vi "THD_MSA_for_teststand_Seq.vi"(6 "Sound_Pressure(dB SPL)":dbl=94.0502, 8 "error in":errorcluster, 9 "Std_Deviation_Thresold":dbl=0.04, 10 "frequency list Input":T6(array[cluster])=[{"frequency [Hz]"=1000.0, "amplitude [V]"=0.373}] {"amplitude [V]" format="%.6f"; "frequency [Hz]" format="%.2f"}, 11 "Peiker_Stepped Sweep Settings":T1={"Input Settings"={"IEPE min time to settle [s]"=0.0, "Responce Channel Settings"={"DSA response channel settings"={"coupling"=10045, "enable IEPE excitation"=FALSE, "IEPE current [mA]"=4.0}, "response channel info"={"sensor sensitivity"=200.0, "engineering units"=2, "dB reference"=2e-05, "custom label"="EU", "weighting filter"=0, "pregain"=0.0}, "AI response settings"={"response channel"="SOUNDACQ/ai1", "max value [V]"=10.0, "min value [V]"=-10.0, "terminal configuration"=-1}}, "Stimulus Channel Settings"={"AI stimulus settings"={"stimulus channel"="SOUNDACQ/ai0", "max value [V]"=10.0, "min value [V]"=-10.0, "terminal configuration"=-1}, "DSA stimulus channel settings"={"coupling"=10045, "enable IEPE excitation"=TRUE, "IEPE current [mA]"=4.0}, "stimulus channel info"={"sensor sensitivity"=11.4, "engineering units"=2, "dB reference"=2e-05, "custom label"="EU", "weighting filter"=0, "pregain"=0.0}}}, "Output Settings"={"AO source settings"={"excitation channel"="SOUNDACQ/ao0", "max value [V]"=10.0, "min value [V]"=-10.0, "terminal configuration"=-1}}} {"Output Settings"."AO source settings"."terminal configuration" items=["Default"=-1, "RSE"=10083, "Differential"=10106, "Pseudodifferential"=12529]; "Output Settings"."AO source settings"."min value [V]" format="%0.2f"; "Output Settings"."AO source settings"."max value [V]" format="%0.2f"; "Input Settings"."Stimulus Channel Settings"."stimulus channel info"."pregain" format="%.2f"; "Input Settings"."Stimulus Channel Settings"."stimulus channel info"."weighting filter" items=["Linear", "A-weighting", "B-weighting", "C-weighting", "ITU-R 468-4", "Dolby", "CCITT", "C-message", "Wb", "Wc", "Wd", "We", "Wf", "Wh", "Wj", "Wk", "Wm", "AES17 20 kHz lowpass", "AES17 40 kHz lowpass", "AES17 20 kHz highpass", "AES17 40 kHz highpass"]; "Input Settings"."Stimulus Channel Settings"."stimulus channel info"."dB reference" format="%^.1e"; "Input Settings"."Stimulus Channel Settings"."stimulus channel info"."engineering units" items=["custom..."=0, "V"=1, "A"=21, "C"=30, "pC"=31, "s"=32, "-"=29, "Pa"=2, "N"=20, "g"=3, "m/s^2"=4, "m/s"=5, "m"=6, "mm/s"=12, "mm"=13, "micron/s"=14, "micron"=15, "in/s^2"=7, "in/s"=8, "in"=9, "mil/s"=10, "mil"=11, "rad/s^2"=16, "rad/s"=17, "rad"=18, "deg/s^2"=26, "deg/s"=27, "deg"=28, "RPM"=22, "cycle/s^2"=23, "Hz"=24, "cycle"=25, "strain"=19]; "Input Settings"."Stimulus Channel Settings"."stimulus channel info"."sensor sensitivity" format="%#_5f"; "Input Settings"."Stimulus Channel Settings"."DSA stimulus channel settings"."IEPE current [mA]" format="%.1f"; "Input Settings"."Stimulus Channel Settings"."DSA stimulus channel settings"."coupling" items=["AC"=10045, "DC"=10050, "GND"=10066]; "Input Settings"."Stimulus Channel Settings"."AI stimulus settings"."terminal configuration" items=["Default"=-1, "RSE"=10083, "NRSE"=10078, "Differential"=10106, "Pseudodifferential"=12529]; "Input Settings"."Stimulus Channel Settings"."AI stimulus settings"."min value [V]" format="%.2f"; "Input Settings"."Stimulus Channel Settings"."AI stimulus settings"."max value [V]" format="%.2f"; "Input Settings"."Responce Channel Settings"."AI response settings"."terminal configuration" items=["Default"=-1, "RSE"=10083, "NRSE"=10078, "Differential"=10106, "Pseudodifferential"=12529]; "Input Settings"."Responce Channel Settings"."AI response settings"."min value [V]" format="%.2f"; "Input Settings"."Responce Channel Settings"."AI response settings"."max value [V]" format="%.2f"; "Input Settings"."Responce Channel Settings"."response channel info"."pregain" format="%.2f"; "Input Settings"."Responce Channel Settings"."response channel info"."weighting filter" items=["Linear", "A-weighting", "B-weighting", "C-weighting", "ITU-R 468-4", "Dolby", "CCITT", "C-message", "Wb", "Wc", "Wd", "We", "Wf", "Wh", "Wj", "Wk", "Wm", "AES17 20 kHz lowpass", "AES17 40 kHz lowpass", "AES17 20 kHz highpass", "AES17 40 kHz highpass"]; "Input Settings"."Responce Channel Settings"."response channel info"."dB reference" format="%^.1e"; "Input Settings"."Responce Channel Settings"."response channel info"."engineering units" items=["custom..."=0, "V"=1, "A"=21, "C"=30, "pC"=31, "s"=32, "-"=29, "Pa"=2, "N"=20, "g"=3, "m/s^2"=4, "m/s"=5, "m"=6, "mm/s"=12, "mm"=13, "micron/s"=14, "micron"=15, "in/s^2"=7, "in/s"=8, "in"=9, "mil/s"=10, "mil"=11, "rad/s^2"=16, "rad/s"=17, "rad"=18, "deg/s^2"=26, "deg/s"=27, "deg"=28, "RPM"=22, "cycle/s^2"=23, "Hz"=24, "cycle"=25, "strain"=19]; "Input Settings"."Responce Channel Settings"."response channel info"."sensor sensitivity" format="%#_5f"; "Input Settings"."Responce Channel Settings"."DSA response channel settings"."IEPE current [mA]" format="%.1f"; "Input Settings"."Responce Channel Settings"."DSA response channel settings"."coupling" items=["AC"=10045, "DC"=10050, "GND"=10066]; "Input Settings"."IEPE min time to settle [s]" format="%.1f"}) -> (0 "error out":errorcluster, 2 "Stimulus Level":cluster{"frequency":dbl[], "magnitude":dbl[]}(graph), 3 "THD-Response":cluster{"frequency":dbl[], "THD":dbl[]}(graph))   [LabVIEW 2018]
doc: "Measures the THD value at a given Frequency and Sound Pressure Level. This VI also shows a pop-up message in case of sound disturbances."
uses:
  Peiker_Stepped Sweep Settings.ctl
  <vilib>/addons/_NISVFA/_Shared subVIs/Controls/svc_DSA Channel Settings.ctl
  <vilib>/addons/_NISVFA/_Shared subVIs/Controls/svc_Channel Info.ctl
  <vilib>/addons/_NISVFA/_Shared subVIs/Controls/svc_Engineering Units Text Ring.ctl
  <vilib>/addons/_NISVFA/_Shared subVIs/Controls/svc_Weighting Filter Text Ring.ctl
panel:
  out "Sensitivity(dB)":dbl=336.0
  in  "Standard_Sensitivity":dbl=94.0502
  out "Meas_Error":bool=TRUE
  out "index":i32=48
  out "THD":dbl=0.5
  out "Sensitivity(mVeff/Pa)":dbl=336.0
  out "Stimulus_Amplitude(Vpeak)":dbl=0.35 min=0.0 format="%.3f"
  in  "stop":bool=TRUE
  out "XY Graph":cluster{dbl[], dbl[]}[](graph)=[{[0.84, 0.944, 1.048, 1.1540000000000001, 1.2590000000000001, 1.3650000000000002, 1.4670000000000003, 1.5720000000000003, 1.6750000000000003, 1.7800000000000002, 1.8880000000000003, 1.9940000000000004, 2.0990000000000006, 2.206000000000001, 2.3080000000000007, 2.412000000000001, 2.520000000000001, 2.626000000000001, 2.733000000000001, 2.836000000000001, 2.942000000000001, 3.048000000000001, 3.154000000000001, 3.2600000000000007, 3.3640000000000008, 3.467000000000001, 3.573000000000001, 3.677000000000001, 3.783000000000001, 3.888000000000001, 3.9930000000000008, 4.099000000000001, 4.201000000000001, 4.307000000000001, 4.412000000000002, 4.517000000000002, 4.6220000000000026, 4.721000000000003, 4.827000000000003, 4.9330000000000025, 5.039000000000002, 5.1430000000000025, 5.248000000000003, 5.354000000000003, 5.461000000000003, 5.568000000000003, 5.674000000000003, 5.780000000000003, 5.885000000000003], [0.5, 0.5, 0.5, 0.5, 0.5, 0.5, 0.5, 0.5, 0.5, 0.5, 0.5, 0.5, 0.5, 0.5, 0.5, 0.5, 0.5, 0.5, 0.5, 0.5, 0.5, 0.5, 0.5, 0.5, 0.5, 0.5, 0.5, 0.5, 0.5, 0.5, 0.5, 0.5, 0.5, 0.5, 0.5, 0.5, 0.5, 0.5, 0.5, 0.5, 0.5, 0.5, 0.5, 0.5, 0.5, 0.5, 0.5, 0.5, 0.5]}, {[0.84, 0.944, 1.048, 1.1540000000000001, 1.2590000000000001, 1.3650000000000002, 1.4670000000000003, 1.5720000000000003, 1.6750000000000003, 1.7800000000000002, 1.8880000000000003, 1.9940000000000004, 2.0990000000000006, 2.206000000000001, 2.3080000000000007, 2.412000000000001, 2.520000000000001, 2.626000000000001, 2.733000000000001, 2.836000000000001, 2.942000000000001, 3.048000000000001, 3.154000000000001, 3.2600000000000007, 3.3640000000000008, 3.467000000000001, 3.573000000000001, 3.677000000000001, 3.783000000000001, 3.888000000000001, 3.9930000000000008, 4.099000000000001, 4.201000000000001, 4.307000000000001, 4.412000000000002, 4.517000000000002, 4.6220000000000026, 4.721000000000003, 4.827000000000003, 4.9330000000000025, 5.039000000000002, 5.1430000000000025, 5.248000000000003, 5.354000000000003, 5.461000000000003, 5.568000000000003, 5.674000000000003, 5.780000000000003, 5.885000000000003], [336.0, 336.0, 336.0, 336.0, 336.0, 336.0, 336.0, 336.0, 336.0, 336.0, 336.0, 336.0, 336.0, 336.0, 336.0, 336.0, 336.0, 336.0, 336.0, 336.0, 336.0, 336.0, 336.0, 336.0, 336.0, 336.0, 336.0, 336.0, 336.0, 336.0, 336.0, 336.0, 336.0, 336.0, 336.0, 336.0, 336.0, 336.0, 336.0, 336.0, 336.0, 336.0, 336.0, 336.0, 336.0, 336.0, 336.0, 336.0, 336.0]}, {[0.84, 0.944, 1.048, 1.1540000000000001, 1.2590000000000001, 1.3650000000000002, 1.4670000000000003, 1.5720000000000003, 1.6750000000000003, 1.7800000000000002, 1.8880000000000003, 1.9940000000000004, 2.0990000000000006, 2.206000000000001, 2.3080000000000007, 2.412000000000001, 2.520000000000001, 2.626000000000001, 2.733000000000001, 2.836000000000001, 2.942000000000001, 3.048000000000001, 3.154000000000001, 3.2600000000000007, 3.3640000000000008, 3.467000000000001, 3.573000000000001, 3.677000000000001, 3.783000000000001, 3.888000000000001, 3.9930000000000008, 4.099000000000001, 4.201000000000001, 4.307000000000001, 4.412000000000002, 4.517000000000002, 4.6220000000000026, 4.721000000000003, 4.827000000000003, 4.9330000000000025, 5.039000000000002, 5.1430000000000025, 5.248000000000003, 5.354000000000003, 5.461000000000003, 5.568000000000003, 5.674000000000003, 5.780000000000003, 5.885000000000003], [0.84, 0.104, 0.104, 0.106, 0.105, 0.106, 0.102, 0.105, 0.103, 0.105, 0.108, 0.106, 0.105, 0.107, 0.102, 0.104, 0.108, 0.106, 0.107, 0.103, 0.106, 0.106, 0.106, 0.106, 0.104, 0.103, 0.106, 0.104, 0.106, 0.105, 0.105, 0.106, 0.102, 0.106, 0.105, 0.105, 0.105, 0.099, 0.106, 0.106, 0.106, 0.104, 0.105, 0.106, 0.107, 0.107, 0.106, 0.106, 0.105]}]
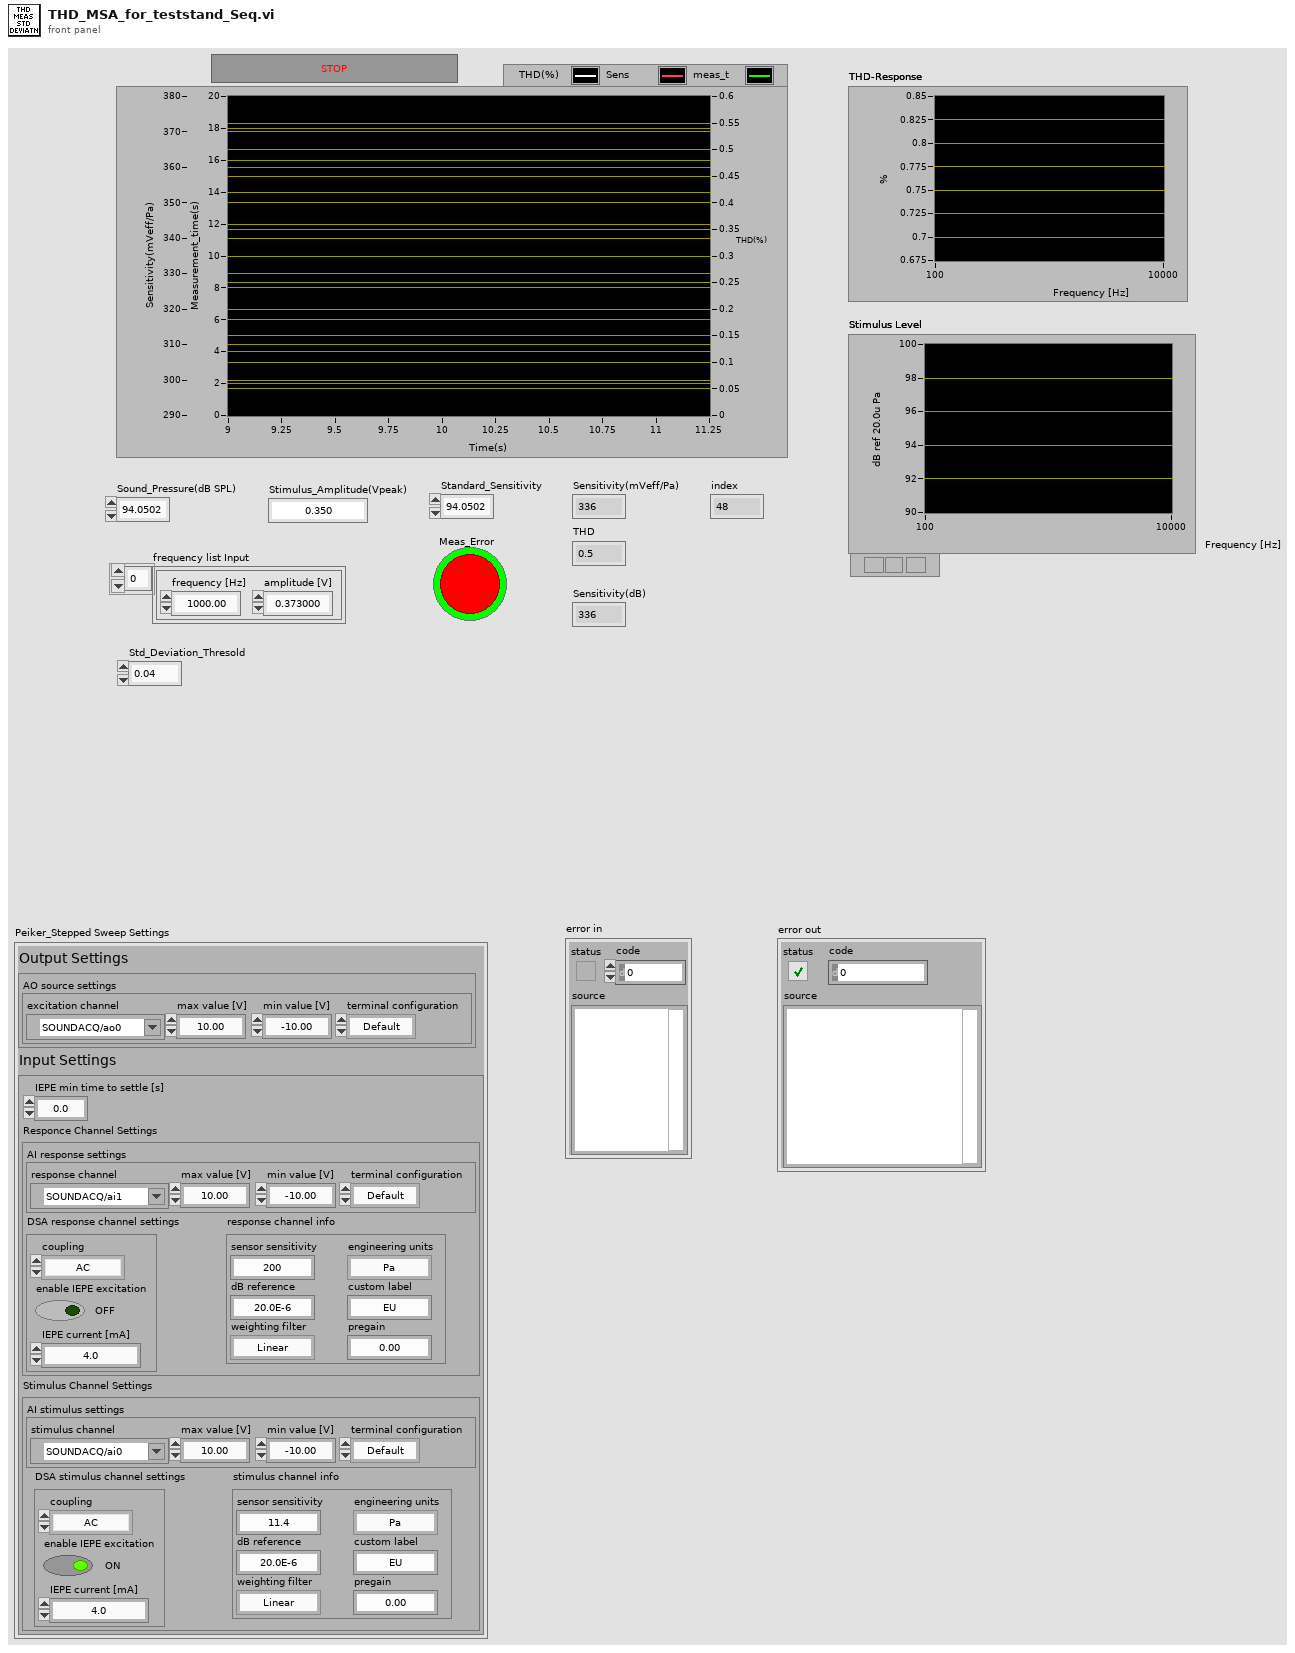
[diagram p1: front panel]
types:
  T1 = typedef "Peiker_Stepped Sweep Settings.ctl" = cluster{"Input Settings":cluster{"IEPE min time to settle [s]":dbl, "Responce Channel Settings":cluster{"DSA response channel settings":T2, "response channel info":T3, "AI response settings":cluster{"response channel":tag, "max value [V]":dbl, "min value [V]":dbl, "terminal configuration":i32}}, "Stimulus Channel Settings":cluster{"AI stimulus settings":cluster{"stimulus channel":tag, "max value [V]":dbl, "min value [V]":dbl, "terminal configuration":i32}, "DSA stimulus channel settings":T2, "stimulus channel info":T3}}, "Output Settings":cluster{"AO source settings":cluster{"excitation channel":tag, "max value [V]":dbl, "min value [V]":dbl, "terminal configuration":i32}}}
  T2 = typedef "svc_DSA Channel Settings.ctl" = cluster{"coupling":i32, "enable IEPE excitation":bool, "IEPE current [mA]":dbl}
  T3 = typedef "svc_Channel Info.ctl" = cluster{"sensor sensitivity":dbl, "engineering units":T4, "dB reference":dbl, "custom label":string, "weighting filter":T5, "pregain":dbl}
  T4 = typedef "svc_Engineering Units Text Ring.ctl" = u16
  T5 = typedef "svc_Weighting Filter Text Ring.ctl" = u16
  T6 = cluster{"frequency [Hz]":dbl, "amplitude [V]":dbl}[]
  T7 = cluster{"frequency [Hz]":dbl, "amplitude [V]":dbl}
  T8 = enum32{"Invalid", "Standard", "Closed", "Hidden", "Minimized", "Maximized"}
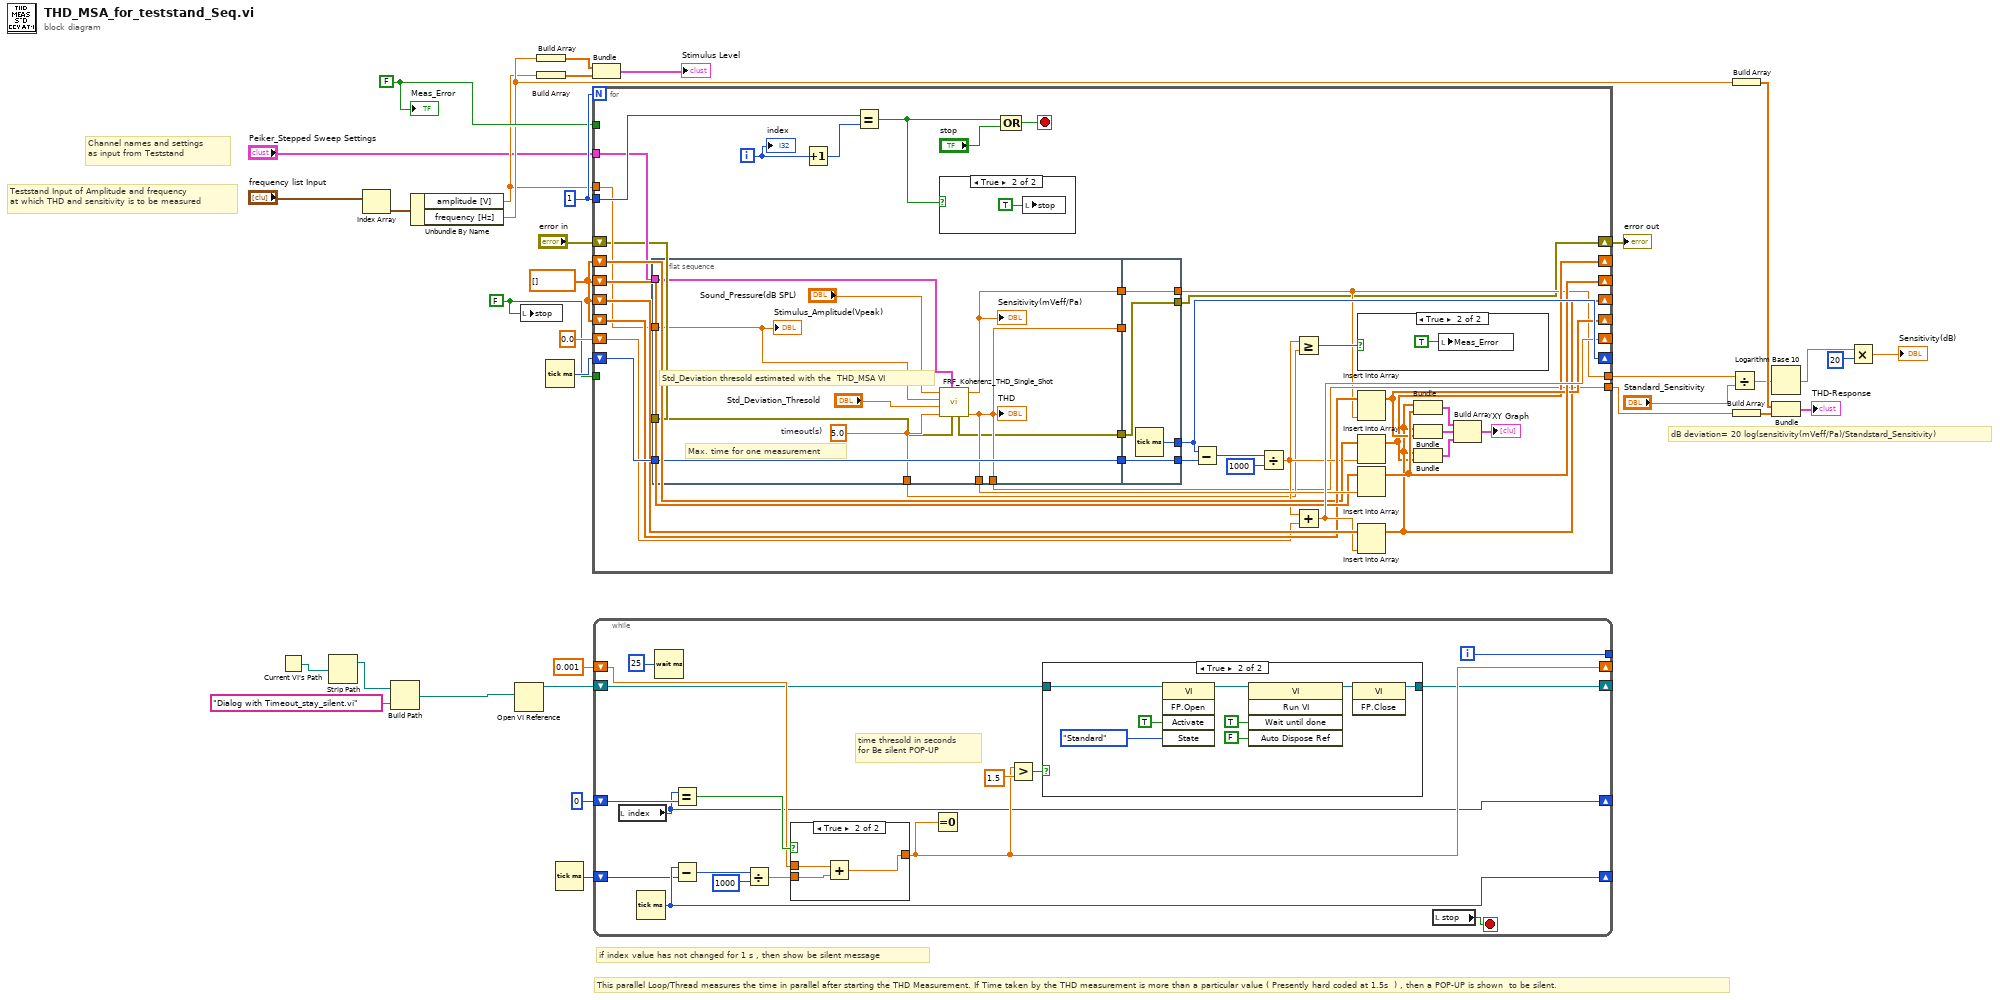
[diagram p0: block diagram]
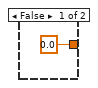
[diagram p3: hidden frame]
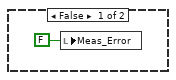
[diagram p4: hidden frame]
diagram:
  w28 = 1 ("Anzahl der Messungen")
  w25 = FALSE ("Meas_Error")
  w29 = FALSE ("stop")
  w26 = dbl[] []
  # "Channel names and settings \nas input from Teststand"
  # "Teststand Input of Amplitude and frequency \nat which THD and sensitivity is to be measured"
  # "This parallel Loop/Thread measures the time in parallel after starting the THD Measurement. If Time taken by the THD measurement is more than a particular value ( Presently hard coded at 1.5s  ) , then a POP-UP is shown  to be silent."
  # "dB deviation= 20 log(sensitivity(mVeff/Pa)/Standstard_Sensitivity)"
  # "if index value has not changed for 1 s , then show be silent message"
  n1 = Current VI's Path() -> (path=w3:path)
  n2 = Strip Path(path=w3) -> (stripped path=w2:path)  [unwired: 1 out]
  n3 = Index Array(array="frequency list Input") -> (element=w23:T7)  [unwired: 1 in]
  n4 = Build Path(base path=w2, name or relative path="Dialog with Timeout_stay_silent.vi") -> (appended path=w1:path)
  n5 = Unbundle By Name(w23) -> ("amplitude [V]"=w14:dbl, "frequency [Hz]"=w15:dbl)
  n6 = Open VI Reference(vi path=w1) -> (vi reference=w27:refnum<vi>)  [unwired: 5 in, 1 out]
  n7 = local write "stop"(w29) -> ()
  n8 = Build Array(w15) -> (w17:dbl[])
  n9 = Build Array(w14) -> (w18:dbl[])
  n10 = Tick Count (ms)() -> (millisecond timer value=w34:u32)
  n11 = Tick Count (ms)() -> (millisecond timer value=w32:u32)
  n12 = Bundle(w17, w18) -> (→"Stimulus Level":cluster{dbl[], dbl[]})  [unwired: 1 in]
  n13 = for {
    N: w28 -> [_]
    shift-right: [w69] -> _
    shift-left: w34 -> [w72]
    shift-right: [w47] -> _
    shift-left: w26 -> [w66]
    shift-right: [w62] -> _
    shift-left: w26 -> [w63]
    shift-right: [w65] -> _
    shift-left: 0.0 -> [w48]
    shift-right: [w56] -> _
    shift-left: w26 -> [w60]
    tunnel: w29 -> [_]
    tunnel: w28 -> [w53]
    shift-right: [w46] -> _
    shift-left: w26 -> [w49]
    tunnel: w25 -> [_]
    tunnel: w14 -> [w41]
    tunnel: [w40] -> w22
    tunnel: [w39] -> w13
    tunnel: "Peiker_Stepped Sweep Settings" -> [w38]
    shift-right: [w36] -> w5
    shift-left: "error in" -> [w35]
    i -> [w55]
    stop <- w51 stop-if-true
    n14 = flat-sequence {
      tunnel: [w80] -> w73
      tunnel: w72 -> [w86]
      tunnel: [w86] -> w70
      tunnel: [w80] -> w64
      tunnel: [w84] -> w61
      tunnel: [w82] -> w42
      tunnel: w41 -> [w81]
      tunnel: [w80] -> w40
      tunnel: w38 -> [w79]
      tunnel: [w78] -> w37
      tunnel: w35 -> [w77]
      tunnel: w73 -> [_]
      tunnel: [w90] -> w69
      tunnel: [w89] -> w71
      tunnel: w70 -> [w89]
      tunnel: [w88] -> w39
      tunnel: w61 -> [w88]
      tunnel: [w87] -> w36
      tunnel: w37 -> [w87]
      frame #0 {
        w82 = 5.0  # timeout(s)
        # "Max. time for one measurement"
        # "Std_Deviation thresold estimated with the  THD_MSA VI"
        n15 = call "FRF_Koherenz_THD_Single_Shot.vi"("error in"=w77, "Peiker_Stepped Sweep Settings"=w79, "timeout(s)"=w82, "Std_Deviation_Thresold"="Std_Deviation_Thresold", "Excitation_amplitude(Vpeak)"=w81, "dB SPL"="Sound_Pressure(dB SPL)") -> ("mean"=w80:dbl, "Sensitivity(mVeff/Pa)"=w84:dbl, "error out"=w78:errorcluster)  [unwired: 3 in]
        "Sensitivity(mVeff/Pa)" <- w84
        "THD" <- w80
        "Stimulus_Amplitude(Vpeak)" <- w81
      }
      frame #1 {
        n16 = Tick Count (ms)() -> (millisecond timer value=w90:u32)
      }
    }
    n17 = Increment(x=w55) -> (x+1=w54:i32)
    n18 = Equal?(x=w53, y=w54) -> (x = y?=w50:bool)
    n19 = case shown="True" w50 {
      frame False {
      }
      frame True {
        n20 = local write "stop"(TRUE ("stop")) -> ()
      }
    }
    n21 = Compound Arithmetic op=OR(w50, "stop") -> (w51:bool)
    n22 = Subtract(x=w69, y=w71) -> (x-y=w68:u32)
    n23 = Divide(x=w68, y=u32 1000) -> (x/y=w44:dbl)
    n24 = Greater Or Equal?(x=w44, y=w42) -> (x >= y?=w43:bool)
    n25 = Add(x=w44, y=w48) -> (x+y=w65:dbl)
    n26 = case shown="True" w43 {
      frame False {
        n27 = local write "Meas_Error"(FALSE ("Meas_Error")) -> ()
      }
      frame True {
        n28 = local write "Meas_Error"(TRUE ("Meas_Error")) -> ()
      }
    }
    n29 = Insert Into Array(array=w60, new element=w39) -> (w56:dbl[])  [unwired: 1 in]
    n30 = Insert Into Array(array=w49, new element=w44) -> (w46:dbl[])  [unwired: 1 in]
    n31 = Insert Into Array(array=w63, new element=w64) -> (w62:dbl[])  [unwired: 1 in]
    n32 = Insert Into Array(array=w66, new element=w65) -> (w47:dbl[])  [unwired: 1 in]
    n33 = Bundle(w47, w62) -> (w59:cluster{dbl[], dbl[]})  [unwired: 1 in]
    n34 = Bundle(w47, w56) -> (w58:cluster{dbl[], dbl[]})  [unwired: 1 in]
    n35 = Bundle(w47, w46) -> (w45:cluster{dbl[], dbl[]})  [unwired: 1 in]
    n36 = Build Array(w59, w58, w45) -> (→"XY Graph":cluster{dbl[], dbl[]}[])
    "index" <- w55
  }
  "error out" <- w5
  n37 = while {
    shift-right: [w95] -> _
    shift-left: 0 ("index") -> [w107]
    shift-right: [w106] -> _
    shift-left: w32 -> [w105]
    shift-right: [w98] -> _
    shift-left: 0.001 -> [w101]
    tunnel: [w94] -> _
    shift-right: [w92] -> _
    shift-left: w27 -> [w93]
    i -> [w94]
    stop <- w97 stop-if-true
    # "time thresold in seconds \nfor Be silent POP-UP"
    n38 = local read "index"() -> (w95:i32)
    n39 = Tick Count (ms)() -> (millisecond timer value=w106:u32)
    n40 = Wait (ms)(milliseconds to wait=u32 25) -> ()  [unwired: 1 out]
    n41 = Equal?(x=w95, y=w107) -> (x = y?=w104:bool)
    n42 = Subtract(x=w106, y=w105) -> (x-y=w103:u32)
    n43 = Divide(x=w103, y=u32 1000) -> (x/y=w100:dbl)
    n44 = case shown="True" w104 {
      tunnel: w101 -> [_ w120]
      tunnel: w100 -> [_ w119]
      tunnel: [0.0 w118] -> w98
      frame False {
      }
      frame True {
        n45 = Add(x=w120, y=w119) -> (x+y=w118:dbl)
      }
    }
    n46 = Equal To 0?(x=w98) -> ()  [unwired: 1 out]
    n47 = Greater?(x=w98, y=1.5) -> (0:w91:bool)
    n48 = case shown="True" w91 {
      tunnel: w93 -> [w108 w112]
      tunnel: [w108 w109] -> w92
      frame False {
      }
      frame True {
        n49 = invoke class="VI" method="FP.Open"(reference=w112, "Activate"=TRUE ("Activate?"), "State"=T8."Standard") -> (reference out=w111:refnum<vi>)  [unwired: 2 in, 4 out]
        n50 = invoke class="VI" method="Run VI"(reference=w111, "Wait until done"=TRUE ("Wait Until Done"), "Auto Dispose Ref"=FALSE ("Auto Dispose Reference")) -> (reference out=w110:refnum<vi>)  [unwired: 2 in, 4 out]
        n51 = invoke class="VI" method="FP.Close"(reference=w110) -> (reference out=w109:refnum<vi>)  [unwired: 2 in, 2 out]
      }
    }
    n52 = local read "stop"() -> (w97:bool)
  }
  n53 = Divide(x=w13, y="Standard_Sensitivity") -> (x/y=w11:dbl)
  n54 = Build Array(w15) -> (w21:dbl[])
  n55 = Build Array(w22) -> (w20:dbl[])
  n56 = Logarithm Base 10(1:w11) -> (0:w10:dbl)
  n57 = Bundle(w21, w20) -> (→"THD-Response":cluster{dbl[], dbl[]})  [unwired: 1 in]
  n58 = Multiply(x=w10, y=20) -> (x*y=→"Sensitivity(dB)":dbl)
  "Meas_Error" <- w25
